vi "FormatList.vi"(0 "values":string[](array[string]), 1 "type":T1) -> (2 "python object":string)   [LabVIEW 2014, in "Python Functions.lvlib"]
uses:
  Python Functions.lvlib
  ListTypesTD.ctl
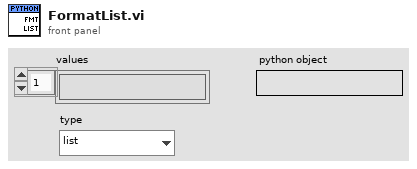
[diagram p1: front panel]
types:
  T1 = typedef "Python Functions.lvlib/ListTypesTD.ctl" = enum16{"list", "tuple", "parameter list", "output list", "return values"}
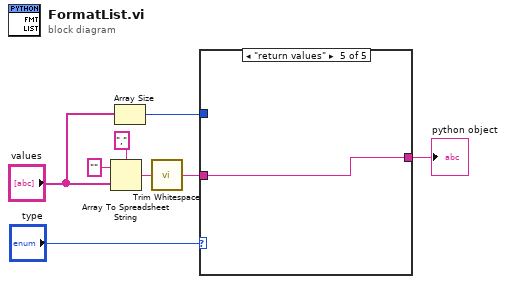
[diagram p0: block diagram]
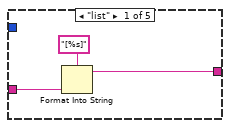
[diagram p2: hidden frame]
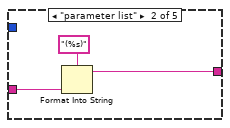
[diagram p3: hidden frame]
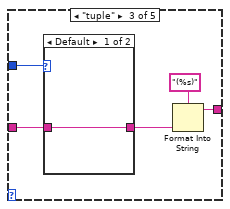
[diagram p4: hidden frame]
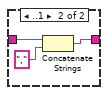
[diagram p5: hidden frame]
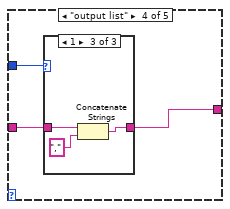
[diagram p6: hidden frame]
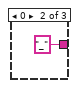
[diagram p8: hidden frame]
diagram:
  n1 = Array To Spreadsheet String(delimiter (Tab)=",", array="values", 3:"" ("format string")) -> (spreadsheet string=w5:string)
  n2 = Array Size(array="values") -> (size(s)=w6:i32)
  n3 = call <vilib>:"Trim Whitespace.vi"("string"=w5) -> ("trimmed string"=w3:string)  [unwired: 1 in]
  n4 = case shown="\"return values\"" "type" {
    tunnel: w6 -> [_ _ w19 w26 _]
    tunnel: w3 -> [w11 w14 w18 w25 w32]
    tunnel: [w9 w12 w16 w24 w32] -> w2
    frame "list" {
      n5 = Format Into String(format string="[%s]", w11) -> (resulting string=w9:string)  [unwired: 2 in, 1 out]
    }
    frame "parameter list" {
      n6 = Format Into String(format string="(%s)", w14) -> (resulting string=w12:string)  [unwired: 2 in, 1 out]
    }
    frame "tuple" {
      n7 = case shown="Default" w19 {
        tunnel: w18 -> [w20 w23]
        tunnel: [w20 w21] -> w15
        frame Default {
        }
        frame ..1 {
          n8 = Concatenate Strings(w23, "," ("string")) -> (w21:string)
        }
      }
      n9 = Format Into String(format string="(%s)", w15) -> (resulting string=w16:string)  [unwired: 2 in, 1 out]
    }
    frame "output list" {
      n10 = case shown="1" w26 {
        tunnel: w25 -> [w27 _ w31]
        tunnel: [w27 "_" ("trimmed string") w29] -> w24
        frame Default {
        }
        frame 0 {
        }
        frame 1 {
          n11 = Concatenate Strings(w31, "," ("string")) -> (w29:string)
        }
      }
    }
    frame "return values" {
    }
  }
  "python object" <- w2
